vi "EMSA SpectralBand.vi"(8 "bandwidth":dbl, 9 "stop frequency":dbl, 10 "start frequency":dbl, 11 "sweep in":cluster{"frequency":dbl[], "amplitude":dbl[]}={"frequency"=array[8000 elements], "amplitude"=array[8000 elements]}) -> (0 "stop index":i32, 1 "start index":i32, 3 "power in band":dbl)   [LabVIEW 2017, in "EmsaAnalysis.lvlib"]
uses:
  <vilib>/addons/InsightCM/Devices/Shared/Emsa/EmsaAnalysis/EmsaAnalysis.lvlib
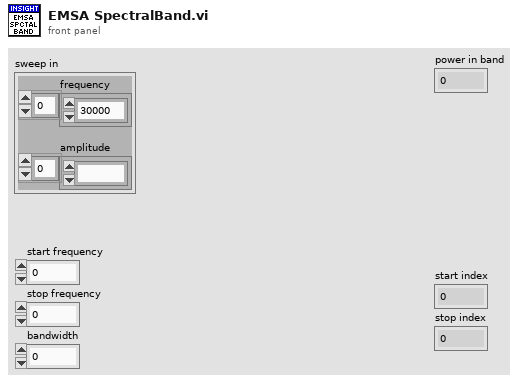
[diagram p1: front panel]
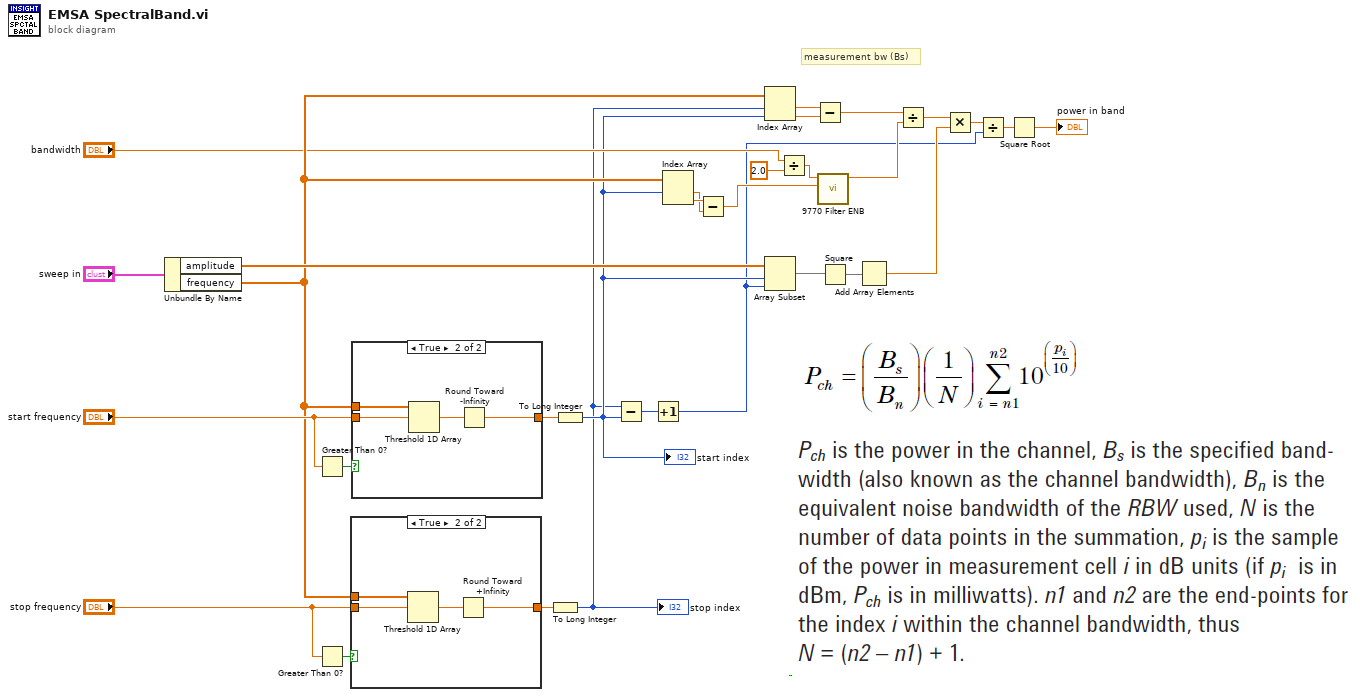
[diagram p0: block diagram]
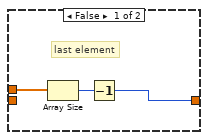
[diagram p2: hidden frame]
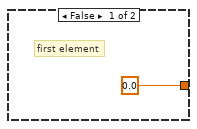
[diagram p3: hidden frame]
diagram:
  # "measurement bw (Bs)"
  n1 = Unbundle By Name("sweep in") -> ("amplitude"=w23:dbl[], "frequency"=w13:dbl[])
  n2 = Greater Than 0?(x="start frequency") -> (x > 0?=w29:bool)
  n3 = Greater Than 0?(x="stop frequency") -> (x > 0?=w27:bool)
  n4 = case shown="True" w27 {
    tunnel: "stop frequency" -> [_ w36]
    tunnel: [w31 w34] -> w4
    tunnel: w13 -> [w33 w37]
    frame False {
      # "last element"
      n5 = Array Size(array=w33) -> (size(s)=w32:i32)
      n6 = Decrement(x=w32) -> (x-1=w31:i32)
    }
    frame True {
      n7 = Threshold 1D Array(2:w36, 3:w37) -> (0:w35:dbl)  [unwired: 1 in]
      n8 = Round Toward +Infinity(x=w35) -> (ceil(x): smallest int >= x=w34:dbl)
    }
  }
  n9 = case shown="True" w29 {
    tunnel: "start frequency" -> [_ w41]
    tunnel: [0.0 w39] -> w6
    tunnel: w13 -> [_ w42]
    frame False {
      # "first element"
    }
    frame True {
      n10 = Threshold 1D Array(2:w41, 3:w42) -> (0:w40:dbl)  [unwired: 1 in]
      n11 = Round Toward -Infinity(1:w40) -> (0:w39:dbl)
    }
  }
  n12 = To Long Integer(number=w4) -> (32bit integer=w3:i32)
  "stop index" <- w3
  n13 = To Long Integer(number=w6) -> (32bit integer=w5:i32)
  "start index" <- w5
  n14 = Subtract(x=w3, y=w5) -> (x-y=w2:i32)
  n15 = Increment(x=w2) -> (x+1=w1:i32)
  n16 = Index Array(array=w13, index #1=w5) -> (element #1=w7:dbl, element #2=w8:dbl)  [unwired: 1 in]
  n17 = Subtract(x=w8, y=w7) -> (x-y=w12:dbl)
  n18 = Index Array(array=w13, index #1=w3, index #2=w5) -> (element #1=w22:dbl, element #2=w21:dbl)
  n19 = Array Subset(array=w23, index=w5, length=w1) -> (w25:dbl[])
  n20 = Divide(x="bandwidth", y=2.0) -> (x/y=w11:dbl)
  n21 = Subtract(x=w22, y=w21) -> (x-y=w20:dbl)
  n22 = call <vilib>:"9770 Filter ENB.vi"("Frequency Spacing"=w12, "Half  BW"=w11) -> ("ENB"=w19:dbl)  [unwired: 9 in]
  n23 = Square(x=w25) -> (x^2=w24:dbl[])
  n24 = Add Array Elements(numeric array=w24) -> (sum=w15:dbl)
  n25 = Divide(x=w20, y=w19) -> (x/y=w16:dbl)
  n26 = Multiply(x=w16, y=w15) -> (x*y=w17:dbl)
  n27 = Divide(x=w17, y=w1) -> (x/y=w18:dbl)
  n28 = Square Root(x=w18) -> (sqrt(x)=→"power in band":dbl)
